vi "2DPoissonInterp.vi"() -> ()   [LabVIEW 2016]
uses:
  <vilib>/Math Plots/3D Math Plots/3D Surface/3D Surface XCtrl/3D Surface.xctl
  <vilib>/gmath/interp.llb/Interpolate 2D (2d X,Y).vi
  <vilib>/Math Plots/3D Math Plots/3D Surface/3D Surface Datatype/Public/Plot Helper (Matrix).vi
  <vilib>/gmath/NI_Gmath.lvlib
  <vilib>/Math Plots/3D Math Plots/3D Surface/3D Surface Datatype/3D Surface Datatype.lvclass
  <vilib>/measure/NI_MABase.lvlib
panel:
  out "Y 2":dbl[](array[numeric])
  out "Y":dbl[](array[numeric])
  in  "ntimes":i32=5
  in  "sampling info 2":cluster{"Fs":dbl, "#s":dbl}={"Fs"=4.0, "#s"=2.0}
  out "Waveform Graph 2":waveform(dbl)(graph)
  in  "sampling info":cluster{"Fs":dbl, "#s":dbl}={"Fs"=4.0, "#s"=2.0}
  out "Waveform Graph":waveform(dbl)(graph)
  out "3D Surface":refnum<class "3D Plot Datatype.lvclass">[](xcontrol)
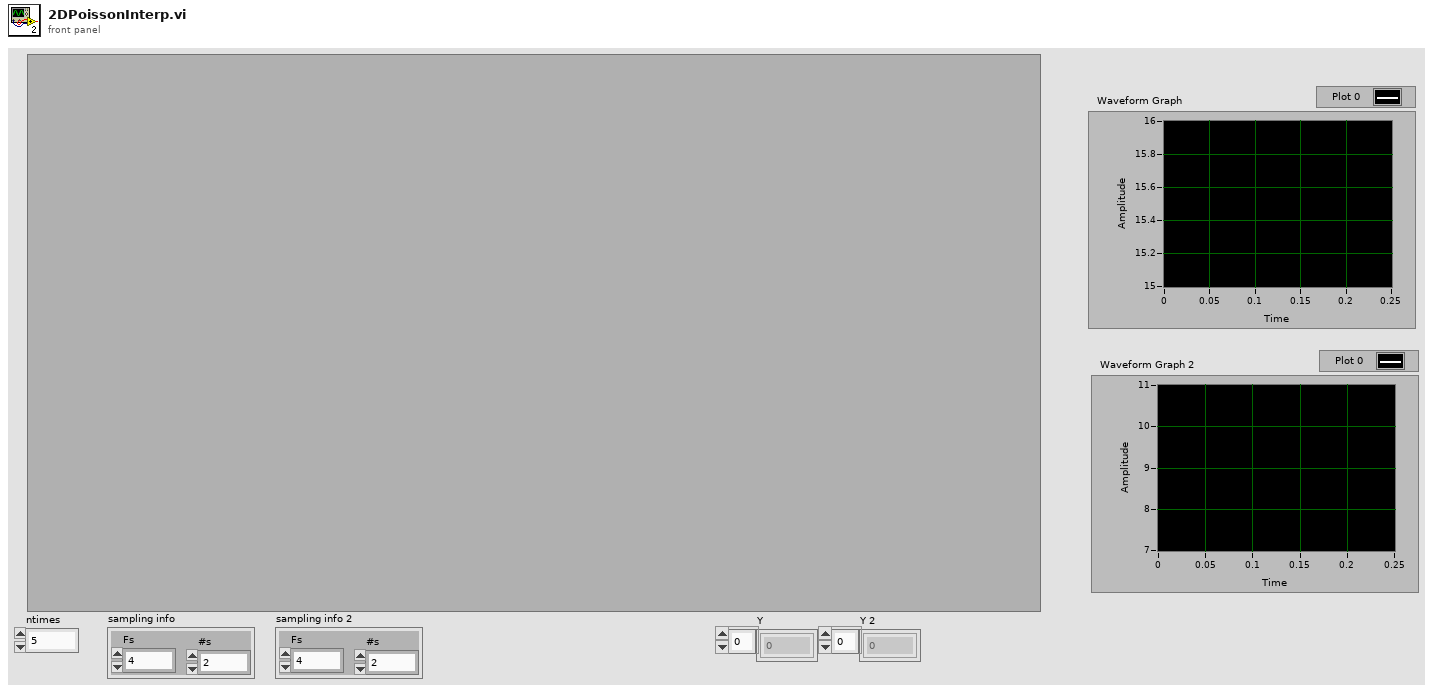
[diagram p1: front panel]
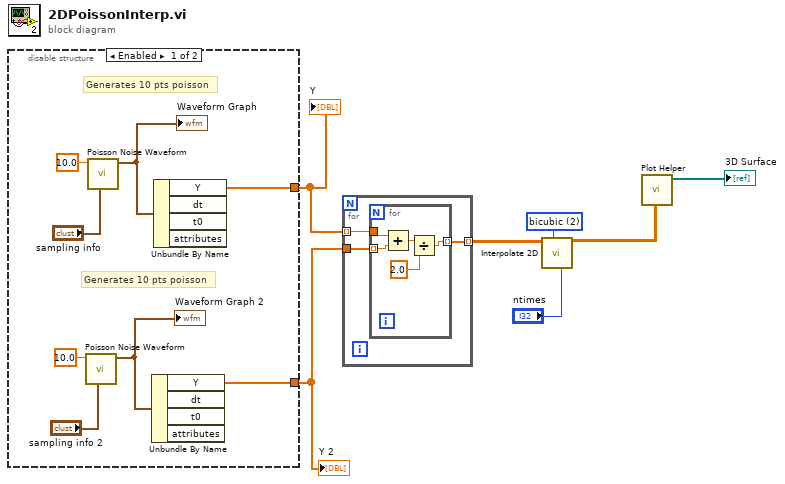
[diagram p0: block diagram]
diagram:
  w2 = 2 items=["nearest", "bilinear", "bicubic", "bicubic spline"] ("method")
  n1 = disable-structure shown="Enabled" {
    disable-tunnel: [w9 _] -> w6
    disable-tunnel: [w8 _] -> w5
    frame Enabled {
      # "Generates 10 pts poisson"
      # "Generates 10 pts poisson"
      n2 = call <vilib>:"Poisson Noise Waveform.vi"("sampling info"="sampling info 2", "mean"=10.0) -> ("signal out"=w11:waveform(dbl))  [unwired: 8 in, 1 out]
      "Waveform Graph 2" <- w11
      n3 = call <vilib>:"Poisson Noise Waveform.vi"("sampling info"="sampling info", "mean"=10.0) -> ("signal out"=w14:waveform(dbl))  [unwired: 8 in, 1 out]
      "Waveform Graph" <- w14
      n4 = Unbundle By Name(w11) -> ("Y"=w8:dbl[])  [unwired: 3 out]
      n5 = Unbundle By Name(w14) -> ("Y"=w9:dbl[])  [unwired: 3 out]
    }
    frame Disabled {
    }
  }
  "Y" <- w6
  "Y 2" <- w5
  n6 = for {
    tunnel: w6 -> [w18] mode=indexing
    tunnel: w5 -> [w17]
    tunnel: [w16] -> w4 mode=indexing
    n7 = for {
      tunnel: w18 -> [w21]
      tunnel: w17 -> [w20] mode=indexing
      tunnel: [w23] -> w16 mode=indexing
      n8 = Add(x=w21, y=w20) -> (x+y=w22:dbl)
      n9 = Divide(x=w22, y=2.0) -> (x/y=w23:dbl)
    }
  }
  n10 = call-poly <vilib>:"Interpolate 2D.vi"("ntimes"="ntimes", "method"=w2, "Z"=w4) -> ("zi"=w3:dbl[][])  [unwired: 5 in, 3 out]
  n11 = call-poly <vilib>:"Plot Helper.vi"("z matrix"=w3) -> ("3D Plot lvclass Array out"=→"3D Surface":refnum<class "3D Plot Datatype.lvclass">[])  [unwired: 5 in, 5 out]
